vi "TRI_Query.vi"(0 "System no.":i32=1 min=1 max=4 step=1, 2 "TriggerIn to query":string[](array[string]), 3 "All triggers?":bool, 5 "error in":errorcluster) -> (14 "Trigger status?":bool[](array[boolean]), 19 "error out":errorcluster)   [LabVIEW 2020]
doc: "Returns the trigger input mode enable status for the given trigger input lines.\n\nE-709: Check controller user manual for available input trigger numbers."
panel:
  # "Returns the trigger input mode enable status for the given \ntrigger input lines."
  # "Query"
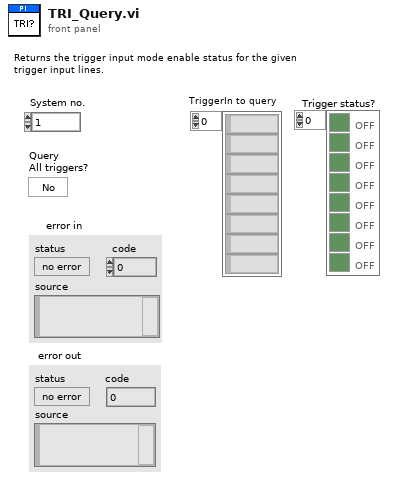
[diagram p1: front panel]
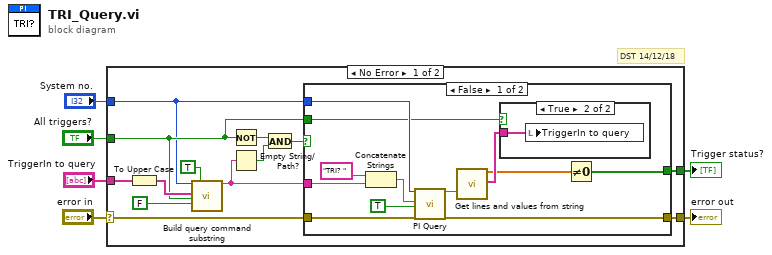
[diagram p0: block diagram]
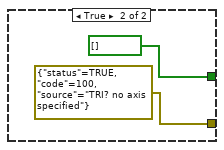
[diagram p3: hidden frame]
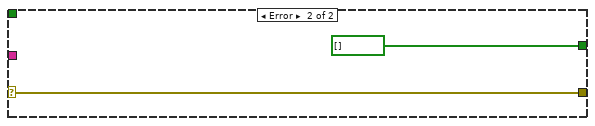
[diagram p4: hidden frame]
diagram:
  # "DST 14/12/18"
  n1 = case shown="No Error" "error in" {
    selector: "error in" -> [w8 w35]
    tunnel: [w13 bool[] [] ("Booleans")] -> w6
    tunnel: "TriggerIn to query" -> [w19 _]
    tunnel: [w18 w35] -> w4
    tunnel: "System no." -> [w7 _]
    tunnel: "All triggers?" -> [w14 _]
    frame No Error {
      n2 = To Upper Case(1:w19) -> (0:w17:string[])
      n3 = call "Build query command substring.vi"("System no."=w7, "Axes to query in"=w17, "Query\nAll axes?"=w14, "For all axes: use\nAxis identifier?"=FALSE ("For all axes: use\nAxis identifier?"), "With space?"=TRUE) -> ("Command substring"=w10:string)  [unwired: 1 in, 13 out]
      n4 = Not(x=w14) -> (.not. x?=w16:bool)
      n5 = Empty String/Path?(string/path=w10) -> (empty?=w9:bool)
      n6 = And(x=w16, y=w9) -> (x .and. y?=w11:bool)
      n7 = case shown="False" w11 {
        tunnel: [w20 errorcluster {"status"=TRUE, "code"=100, "source"="TRI? no axis specified"} ("error out")] -> w18
        tunnel: w10 -> [w28 _]
        tunnel: w7 -> [w27 _]
        tunnel: w8 -> [w26 _]
        tunnel: w14 -> [w25 _]
        tunnel: [w22 bool[] []] -> w13
        frame False {
          n8 = Concatenate Strings("TRI? ", w28) -> (w29:string)
          n9 = call "PI Query.vi"("System no."=w27, "String to send"=w29, "Attach termination char.?"=TRUE ("Attach Linefeed?"), "error in"=w26) -> ("String read"=w21:string, "error out"=w20:errorcluster)  [unwired: 3 in, 11 out]
          n10 = call "Get lines and values from string.vi"("Input string"=w21) -> ("Numerical values"=w23:dbl[], "Item name"=w24:string[])  [unwired: 1 in, 16 out]
          n11 = case shown="True" w25 {
            tunnel: w24 -> [_ w32]
            frame False {
            }
            frame True {
              n12 = local write "TriggerIn to query"(w32) -> ()
            }
          }
          n13 = Not Equal To 0?(x=w23) -> (x != 0?=w22:bool[])
        }
        frame True {
        }
      }
    }
    frame Error {
    }
  }
  "error out" <- w4
  "Trigger status?" <- w6
